vi "PH_Sequencer.SCR Open Rods.vi"(0 "i ref in":refnum<vi>, 5 "error in (no error)":errorcluster) -> (14 "i ref out":refnum<vi>, 19 "error out":errorcluster)   [LabVIEW 2014, in "PH_Sequencer.lvlib"]
doc: "This VI sends a state change request to the Seq SM. If the sequencer is in state \"Start PPMA\", and all PPMA PUs which are in use are in state PU SM \"Open Dump Rods\", \"Open Rods\" is requested."
uses:
  PH_Sequencer.lvlib
  PH_Basics/PH_PP_Common/PH_PP_Common.PUs.ctl
  PH_Basics/PH_PowerUnit_BaseClass/PH_PowerUnit_BaseClass.SM States.ctl
  CS_Core/BaseSM/BaseSM.lvlib
  PH_BeamlineInformation/PH_BeamlineInformation.lvlib
  PH_Basics/PH_PP_Common/PH_PP_Common.lvlib
  PH_Basics/PH_PowerUnit_BaseClass/PH_PowerUnit_BaseClass.lvlib
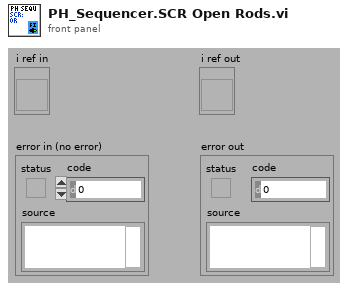
[diagram p1: front panel]
types:
  T1 = typedef "PH_PowerUnit_BaseClass.lvlib/PH_PowerUnit_BaseClass.SM States.ctl" = enum16{".", "Stand by", "Switch PU on", "Configure", "Set Default Voltage", "Set STANDBY", "Set READY", "Wait for Shot Cmd", "Open Dump Rods", "Open Ross Relais", "Close Ross Relais", "Switch PSU on", "Switch PSU off", "Charge", "Switch GD Channel on", "Close Dump Rods", "Rods-TO", "RR-TO", "PSU-TO", "Trigger-TO"}
  T2 = typedef "PH_PP_Common.lvlib/PH_PP_Common.PUs.ctl" = enum16{"no Info", "PA-19mm-1", "PA-19mm-2", "PA-45mm-PILC", "PA-45mm-MAIN", "MA-PU-1", "MA-PU-2", "MA-PU-3", "MA-PU-4", "MA-PU-5", "MA-PU-6", "MA-FR", "MA-PILC", "PA-45mm-DP"}
  T3 = typedef "PH_Sequencer.lvlib/PH_Sequencer.i attribute.ctl" = cluster{"GUI Refs":cluster{"Main Off":refnum<vi>, "Fire":refnum<vi>, "Status":refnum<vi>, "Ready":refnum<vi>, "Waiting Time":refnum<vi>, "Timeout":refnum<vi>, "PPMA Ready":refnum<vi>, "Sequencer SM State":refnum<vi>, "PPPA Ready":refnum<vi>, "Calorimeter":refnum<vi>, "Beamline Ready":refnum<vi>, "Clear Beamline":refnum<vi>, "Linkage PPMA Rods":refnum<vi>, "Linkage Current PA":refnum<vi>, "Linkage Current MA":refnum<vi>, "Timing Ready":refnum<vi>, "State Timing":refnum<vi>, "Force Timing":refnum<vi>, "PSDB Shot Comment":refnum<vi>, "State PA Backreflection":refnum<vi>, "Beamline Z6 Ready":refnum<vi>, "Clear Z6 Beamline":refnum<vi>, "Sequence length":refnum<vi>, "Timing Mode":refnum<vi>, "Slow Trigger Settings":refnum<vi>, "Experiment Description":refnum<vi>, "State PSDB":refnum<vi>, "PSDB Ready":refnum<vi>, "Set PSDB Settings":refnum<vi>, "Get PSDB Info":refnum<vi>, "Take Snapshot":refnum<vi>, "Shottype":refnum<vi>, "Experiment":refnum<vi>, "Phase Frontends":refnum<vi>, "PP 45mm PILC in use":refnum<vi>}, "Status Info":cluster{"Machine Status":T4, "WaitingTime":i32, "Timeout":bool}, "Readyness":cluster{"Ready to shot":bool, "PPMA Ready":bool, "PPPA Ready":bool, "BL Ready":bool, "Timing Ready":bool, "BL Z6 Ready":bool, "PSDBReady":bool}, "Instancenames":cluster{"PPMA Rods":string, "PP Current Meas":string, "PH Beamline Chief":string, "PA Backrefl Meas":string, "Z6 Beamline Chief":string}, "Data to read":bool, "Calorimeter":cluster{"Instancename":string, "On":bool, "linked":bool}, "Linkage":cluster{"PPMA Rods":bool, "PP Current Meas":bool, "PHELIX Beamline Chief":bool, "PA Backrefl Meas":bool, "Z6 Beamline Chief":bool}, "Timing":cluster{"Instance":string, "linked":bool, "Status":T4, "Timing Mode":T5, "Slow Trigger Settings":T6, "Info available":cluster{"ext SlowTrigger":bool, "T2":bool, "Mode":bool, "Delay Slow Trigger":bool, "Phase FEs":bool}, "FE Phase":T7}, "Service ID R2S":i32, "PSDB":cluster{"Controller Instance":string, "Controller Status":T4, "Controller linked":bool, "Settings acknowledged":bool, "Current Experiment ID":i16, "Current Shot Type":i16, "Current Comment":string, "Remember Settings":bool, "Write 2 early":bool}, "PSDB Data":cluster{"Main Off?":bool, "Sequence Length":dbl, "Sequence startet":timestamp}, "6P 4Q Positions":cluster{"Instancename":string, "linked":bool, "Position":T8}[], "PUs":T9[]}
  T4 = typedef "PH_StatusHandler.lvlib/PH_StatusHandler.Status.ctl" = i16
  T5 = typedef "PH_Timing.lvlib/PH_Timing.Timing Mode.ctl" = cluster{"T2":i16, "Modeselector":enum32{"10 Hz", "0.5 Hz", "Shot"}}
  T6 = typedef "PH_Timing.lvlib/PH_Timing.Slow Trigger Settings.ctl" = cluster{"Delay":dbl, "externally triggered?":bool}
  T7 = typedef "PH_Timing.lvlib/PH_Timing.Phase FEs.ctl" = cluster{"Phase":dbl}
  T8 = typedef "PH_4_Pos_Selector.lvlib/PH_4_Pos_Selector.Position Selector.ctl" = u16
  T9 = typedef "PH_Sequencer.lvlib/PH_Sequencer.Head.ctl" = cluster{"PowerUnit":T2, "GUI Ref":refnum<vi>, "Information":T10, "linked?":bool, "GUI Ref Current Voltage":refnum<vi>}
  T10 = typedef "PH_Sequencer.lvlib/PH_Sequencer.PU Information.ctl" = cluster{"State":T4, "Waiting Time [s]":dbl, "PU State SM":T1, "PU Timeout SM":T1}
  T11 = typedef "PH_BeamlineInformation.lvlib/PH_BeamlineInformation.i attribute.ctl" = cluster{"BL GUI Elements of Services":cluster{"Service Name":string, "GUI Elements":refnum<vi>[], "Status":i32}[], "Powermeters":T12, "Efficiency":T13, "Heads":T14[]}
  T12 = typedef "PH_BeamlineInformation.lvlib/PH_BeamlineInformation.Powermeter.ctl" = cluster{"ns FE":cluster{"GUI Ref":refnum<vi>, "Value":dbl}, "fs FE":cluster{"GUI Ref":refnum<vi>, "Value":dbl}, "PA":cluster{"GUI Ref":refnum<vi>, "Value":dbl}, "MA":cluster{"GUI Ref":refnum<vi>, "Value":dbl}, "Z6 green":cluster{"GUI Ref":refnum<vi>, "Value":dbl}, "Z6 IR":cluster{"GUI Ref":refnum<vi>, "Value":dbl}, "Z6 COS":cluster{"GUI Ref":refnum<vi>, "Value":dbl}}
  T13 = typedef "PH_BeamlineInformation.lvlib/PH_BeamlineInformation.Efficiency.ctl" = cluster{"PA Gain":cluster{"GUI Ref":refnum<vi>, "Value":dbl}, "MA Gain":cluster{"GUI Ref":refnum<vi>, "Value":dbl}, "Z6 green Conversion":cluster{"GUI Ref":refnum<vi>, "Value":dbl}, "Z6 Comp Losses":cluster{"GUI Ref":refnum<vi>, "Value":dbl}}
  T14 = typedef "PH_BeamlineInformation.lvlib/PH_BeamlineInformation.Head.ctl" = cluster{"PowerUnit":T2, "in use":cluster{"Value":bool, "GUI Ref":refnum<vi>, "linked":bool}, "voltage":cluster{"Value":dbl, "GUI Ref":refnum<vi>, "linked":bool}}
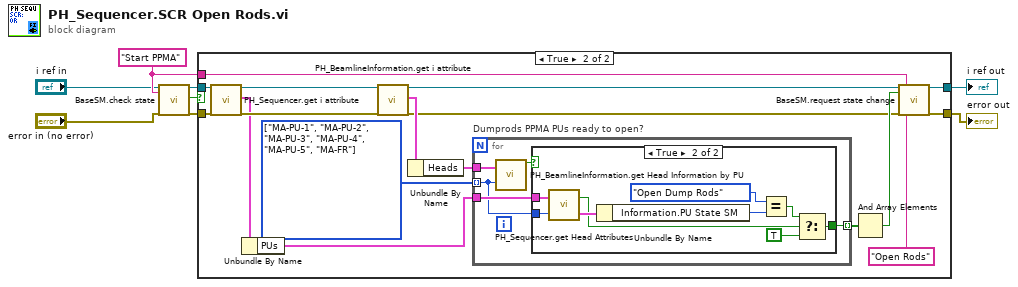
[diagram p0: block diagram]
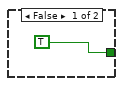
[diagram p3: hidden frame]
diagram:
  w8 = "Start PPMA" ("requested state")
  n1 = call "BaseSM.check state.vi"("i ref in"="i ref in", "requestedState"=w8, "error in (no error)"="error in (no error)") -> ("i ref out"=w2:refnum<vi>, "OK"=w1:bool, "error out"=w3:errorcluster)  [unwired: 11 in, 3 out]
  n2 = case shown="True" w1 {
    tunnel: w8 -> [_ w27]
    tunnel: [w9 w25] -> w7
    tunnel: [w10 w24] -> w6
    tunnel: w3 -> [w9 w21]
    tunnel: w2 -> [w10 w19]
    frame False {
    }
    frame True {
      w14 = T2[] [enum."MA-PU-1", enum."MA-PU-2", enum."MA-PU-3", enum."MA-PU-4", enum."MA-PU-5", enum."MA-FR"] items=["no Info", "PA-19mm-1", "PA-19mm-2", "PA-45mm-PILC", "PA-45mm-MAIN", "MA-PU-1", "MA-PU-2", "MA-PU-3", "MA-PU-4", "MA-PU-5", "MA-PU-6", "MA-FR", "MA-PILC", "PA-45mm-DP"]
      n3 = call "PH_Sequencer.get i attribute.vi"("i ref in"=w19, "error in (no error)"=w21) -> ("i ref out"=w18:refnum<vi>, "i attribute"=w17:T3, "error out"=w20:errorcluster)  [unwired: 15 in]
      n4 = Unbundle By Name(w17) -> ("PUs"=w13:T9[])
      n5 = call "PH_BeamlineInformation.get i attribute.vi"("i ref in"=w18, "error in (no error)"=w20) -> ("i ref out"=w16:refnum<vi>, "i attribute"=w22:T11, "error out"=w15:errorcluster)  [unwired: 15 in]
      n6 = Unbundle By Name(w22) -> ("Heads"=w11:T14[])
      n7 = for "Dumprods PPMA PUs ready to open?" {
        tunnel: [w32] -> w12 mode=indexing
        tunnel: w13 -> [w31]
        tunnel: w14 -> [w29] mode=indexing
        tunnel: w11 -> [w28]
        n8 = call "PH_BeamlineInformation.get Head Information by PU.vi"("Heads"=w28, "Power Unit"=w29) -> ("In Use?"=w30:bool)  [unwired: 12 in, 5 out]
        n9 = case shown="True" w30 {
          tunnel: [TRUE w41] -> w32
          tunnel: w29 -> [_ w39]
          tunnel: w31 -> [_ w40]
          frame False {
          }
          frame True {
            n10 = call "PH_Sequencer.get Head Attributes.vi"("PowerUnit"=w39, "Heads"=w40) -> ("Head"=w38:T9, "Head found?"=w37:bool)
            n11 = Unbundle By Name(w38) -> ("Information.PU State SM"=w36:T1)
            n12 = Equal?(x=PH_PowerUnit_BaseClass.SM_States."Open Dump Rods", y=w36) -> (x = y?=w35:bool)
            n13 = Select(t=w35, s=w37, f=TRUE) -> (s? t:f=w41:bool)
          }
        }
      }
      n14 = And Array Elements(Boolean array=w12) -> (logical AND=w23:bool)
      n15 = call "BaseSM.request state change.vi"("i ref in"=w16, "change"=w23, "error in (no error)"=w15, "allowed current state"=w27, "requested state"="Open Rods" ("next state")) -> ("i ref out"=w24:refnum<vi>, "error out"=w25:errorcluster)  [unwired: 11 in, 2 out]
    }
  }
  "error out" <- w7
  "i ref out" <- w6
